vi "Voltage against time loop.vi"() -> ()   [LabVIEW 2015]
doc: "This example VI shows how to convert string data elements to numeric elements so it can be graphed and displayed on an XY Graph."
uses:
  <instrlib>/Keithley 27XX/Public/Data/Read Multiple Direct.vi
  <instrlib>/Keithley 27XX/Keithley 27XX.lvlib
panel:
  out "concatenated string":string
  out "XY Graph":T1(graph)
  in  "file (use dialog)":path=path "C:/Users/Guest_2/Desktop/Zong Long/Data trial.txt"
  in  "Function (6: Temp)":u16(ring)=6 items=["DC Voltage", "AC Voltage", "DC Current", "AC Current", "Resistance", "Four-Wire Resistance", "Temperature (C)", "Frequency", "Period", "Continuity"]
  in  "Sample Count (10)":i32=10
  in  "Channel List (101)":string="101"
  in  "Serial Configuration":T2={"Baud Rate (9600)"=9600, "Flow Control (1: XON/XOFF)"=1, "Termination Char (0:CR)"=0} {"Termination Char (0:CR)" items=["CR", "LF", "CRLF (Do not use)", "LFCR (Do not use)"]; "Flow Control (1: XON/XOFF)" items=["None", "XON/XOFF", "RTS/CTS (2701 Only)", "XON/XOFF & RTS/CTS (2701 Only)"]; "Baud Rate (9600)" items=["300"=300, "600"=600, "1200"=1200, "2400"=2400, "4800"=4800, "9600"=9600, "19.2k"=19200, "38.4k (2701 Only)"=38400, "57.6k (2701 Only)"=57600, "115.2k (2701 Only)"=115200]}
  in  "Timeout (30000 milliseconds)":u32=30000
  in  "VISA resource name":refnum<visa-resource-name>="GPIB0::19::INSTR"
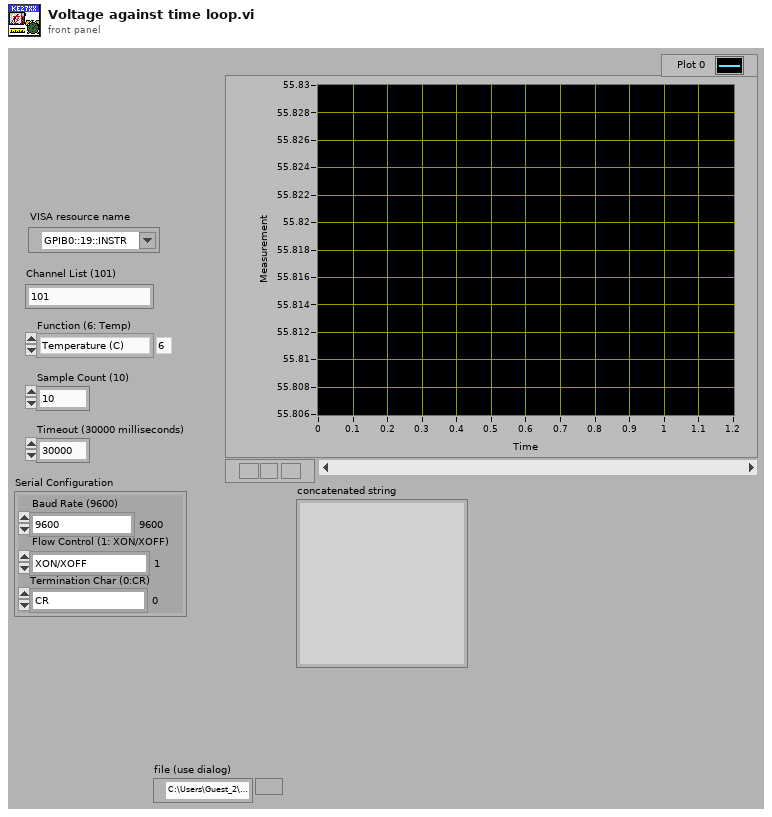
[diagram p1: front panel]
types:
  T1 = cluster{"Measurement Data":dbl[], "Converted Numeric Array":dbl[]}
  T2 = cluster{"Baud Rate (9600)":u32, "Flow Control (1: XON/XOFF)":u16, "Termination Char (0:CR)":u16}
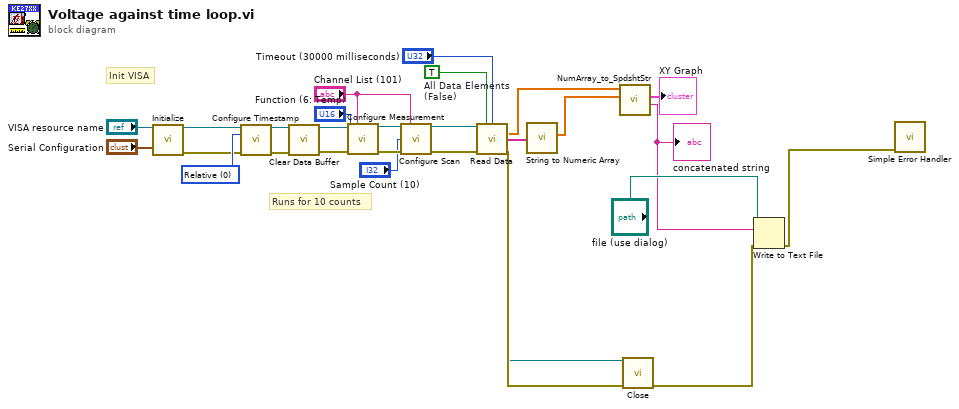
[diagram p0: block diagram]
diagram:
  w17 = u16 0 items=["Relative", "Real Time Clock"] ("Timestamp Type (0: Relative)")
  w27 = TRUE  # All Data Elements (False)
  # "Runs for 10 counts"
  # "Init VISA"
  n1 = call <instrlib>:"Initialize.vi"("VISA resource name"="VISA resource name", "Serial Configuration"="Serial Configuration") -> ("VISA resource name out"=w14:refnum<visa-resource-name>, "error out"=w13:errorcluster)  [unwired: 12 in]
  n2 = call <instrlib>:"Configure Timestamp.vi"("VISA resource name"=w14, "Timestamp Type (0: Relative)"=w17, "error in (no error)"=w13) -> ("VISA resource name out"=w19:refnum<visa-resource-name>, "error out"=w18:errorcluster)  [unwired: 11 in]
  n3 = call <instrlib>:"Clear Data Buffer.vi"("VISA resource name"=w19, "error in (no error)"=w18) -> ("VISA resource name out"=w16:refnum<visa-resource-name>, "error out"=w20:errorcluster)  [unwired: 12 in]
  n4 = call <instrlib>:"Configure Measurement.vi"("VISA resource name"=w16, "Scan List (Empty)"="Channel List (101)", "Function (0: DC Voltage)"="Function (6: Temp)", "error in (no error)"=w20) -> ("VISA resource name out"=w24:refnum<visa-resource-name>, "error out"=w22:errorcluster)  [unwired: 10 in]
  n5 = call <instrlib>:"Configure Scan.vi"("VISA resource name"=w24, "Channel List (101:110)"="Channel List (101)", "Sample Count (100)"="Sample Count (10)", "error in (no error)"=w22) -> ("VISA resource name out"=w12:refnum<visa-resource-name>, "error out"=w11:errorcluster)  [unwired: 10 in]
  n6 = call-poly <instrlib>:"Read Data.vi"("VISA resource name"=w12, "All Data Elements (False)"=w27, "Timeout (30000 milliseconds)"="Timeout (30000 milliseconds)", "error in (no error)"=w11) -> ("VISA resource name out"=w8:refnum<visa-resource-name>, "Measurement Data"=w4:dbl[], "Time Stamp"=w10:string[], "error out"=w9:errorcluster)  [unwired: 6 in, 2 out]
  n7 = call <instrlib>:"String to Numeric Array.vi"("String Array"=w10) -> ("Numeric Array"=w3:dbl[])  [unwired: 10 in]
  n8 = call "NumArray_to_SpdshtStr.vi"("element 2"=w3, "element"=w4) -> ("concatenated string"=w2:string, "XY Graph"=→"XY Graph":T1)  [unwired: 8 in]
  "concatenated string" <- w2
  n9 = call <instrlib>:"Close.vi"("VISA resource name"=w8, "error in (no error)"=w9) -> ("error out"=w5:errorcluster)  [unwired: 13 in]
  n10 = Write to Text File(file (use dialog)="file (use dialog)", text=w2, error in=w5) -> (error out=w6:errorcluster)  [unwired: 1 in, 2 out]
  n11 = call <vilib>:"Simple Error Handler.vi"("error in (no error)"=w6) -> ()  [unwired: 4 in, 5 out]
